vi "Write Dispatcher Response.vi"(6 "overwrite on timeout (T)":bool, 8 "error in (no error)":errorcluster, 9 "timeout in ms (0)":i32 format="%d ms", 10 "response":T1, 11 "Dispatcher Interface in":refnum<class "Dispatcher Interface.lvclass">) -> (0 "error out":errorcluster, 3 "Dispatcher Interface out":refnum<class "Dispatcher Interface.lvclass">)   [LabVIEW 2017, in "DSF Core.lvlib" / "Dispatcher Interface.lvclass"]
uses:
  Dispatcher Interface.lvclass
  C:/Git/DSF/Data Sharing Framework/Source/Core/Engine/Classes/Interfaces/Interface/Interface.lvclass
  Response Data.ctl
  Response.ctl
  Parameters.ctl
  Interface/RT FIFO Data.ctl
  Interface/RT FIFO Parameters.ctl
  Interface/Interface.lvclass/Interface.ctl
  Interface/Write RT FIFO.vi
  Response Timeout.vi
  Interface/Interface.lvclass
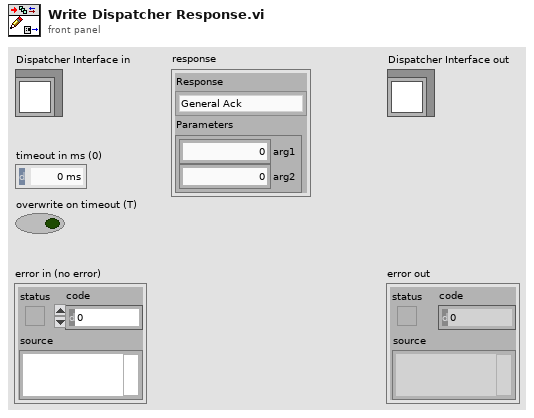
[diagram p1: front panel]
types:
  T1 = typedef "DSF Core.lvlib/Dispatcher Interface.lvclass/Response Data.ctl" = cluster{"Response":T2, "Parameters":T3}
  T2 = typedef "DSF Core.lvlib/Dispatcher Interface.lvclass/Response.ctl" = enum8{"General Ack", "Error", "Shutting Down"}
  T3 = typedef "DSF Core.lvlib/Dispatcher Interface.lvclass/Parameters.ctl" = cluster{"arg1":u64, "arg2":u64}
  T4 = typedef "DSF Core.lvlib/Interface.lvclass/RT FIFO Data.ctl" = cluster{"Command":u8, "Payload":T5}
  T5 = typedef "DSF Core.lvlib/Interface.lvclass/RT FIFO Parameters.ctl" = cluster{"arg1":u64, "arg2":u64}
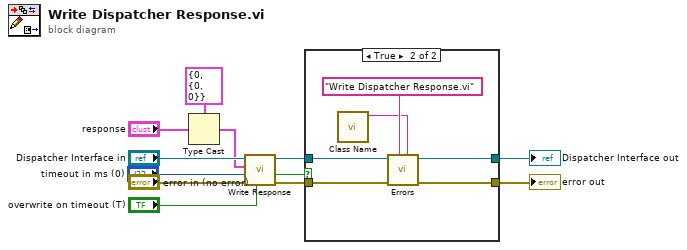
[diagram p0: block diagram]
diagram:
  n1 = Type Cast(type=T4 {"Command"=0, "Payload"={"arg1"=0, "arg2"=0}} ("element"), x="response") -> (*(type *) &x=w7:T4)
  n2 = call "Write Response.vi"("overwrite on timeout (T)"="overwrite on timeout (T)", "error in (no error)"="error in (no error)", "timeout in ms (0)"="timeout in ms (0)", "response"=w7, "Interface in"="Dispatcher Interface in") -> ("error out"=w4:errorcluster, "timed out?"=w3:bool, "Interface out"=w5:refnum<class "Dispatcher Interface.lvclass">)  [unwired: 4 in]
  n3 = case shown="True" w3 {
    tunnel: w4 -> [w13 w18]
    tunnel: w5 -> [w14 w19]
    tunnel: [w14 w17] -> w2
    tunnel: [w13 w16] -> w1
    frame False {
    }
    frame True {
      n4 = call "Class Name.vi"() -> ("class name"=w15:string)  [unwired: 11 in]
      n5 = call-poly "Errors.vi"("error source class name"=w15, "error source vi name"="Write Dispatcher Response.vi", "error in (no error)"=w18, "Interface in"=w19) -> ("error out"=w16:errorcluster, "Interface out"=w17:refnum<class "Dispatcher Interface.lvclass">)  [unwired: 6 in]
    }
  }
  "error out" <- w1
  "Dispatcher Interface out" <- w2
